vi "Main Page.vi"(8 "error in (no error)":errorcluster, 11 "Node Ptr":T1 format="%.0x") -> (0 "error out":errorcluster)   [LabVIEW 2019, in "MD4Logger System Explorer.lvlib"]
uses:
  MD4Logger System Explorer.lvlib
  <vilib>/NI VeriStand/Custom Device API/Custom Device Item Ref.ctl
  <vilib>/NI VeriStand/Custom Device API/Custom Device Channel.ctl
  <vilib>/NI VeriStand/Custom Device API/Custom Device Channel Type.ctl
  Shared/Constants.vi
  <vilib>/NI VeriStand/Custom Device API/Get Item Property (Path).vi
  <vilib>/NI VeriStand/Custom Device API/Get Item Property (String).vi
  <vilib>/NI VeriStand/Custom Device Tools/Custom Device Utility Library/NI VeriStand - Search for Item by GUID.vi
  <vilib>/NI VeriStand/Custom Device API/Set Item Property (String).vi
  <vilib>/NI VeriStand/Custom Device API/Set Item Property (Path).vi
  <vilib>/NI VeriStand/Custom Device API/Custom Device API.lvlib
  <vilib>/NI VeriStand/Custom Device Tools/Custom Device Utility Library/Custom Device Utility Library.lvlib
  Shared/MD4Logger Shared.lvlib
panel:
  in  "File Name":string
  in  "Channel Unit":string
  in  "MDF4 Folder Path":path
  in  "Add":bool
  in  "Channel Name":string
  out "Version":string
  in  "Specific Header":cluster{"Section Name":string}={"Section Name"="Custom Device Item Settings"}
  in  "General Header":cluster{"Section Name":string}={"Section Name"="General Custom Device Settings"}
  in  "Description":string
  in  "Name":string
  # "STEPS\n\nConfiguration\n1. Set the folder path where the MDF4 files should be logged and set the FileName.\n2. Set the Channel Name and Unit and click Add Channel to create MDF4 channels.\n\nRunning\n1. Create New File by setting Command CreateFile to 1\n2. Enable StartLogging by setting Command StartLogging to 1"
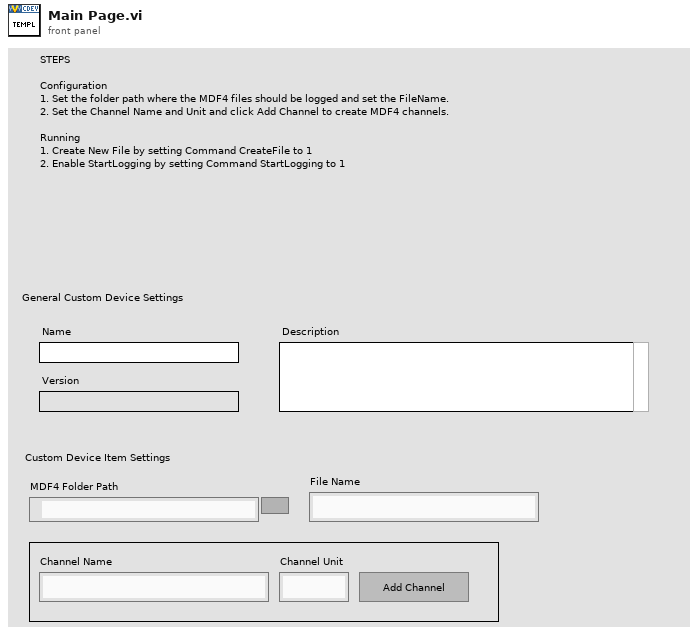
[diagram p1: front panel]
types:
  T1 = typedef "Custom Device API.lvlib/Custom Device Item Ref.ctl" = u64
  T2 = typedef "Custom Device API.lvlib/Custom Device Item Info.ctl" = cluster{"Name":string, "Is Channel":bool, "GUID":string, "Is Waveform":bool}
  T3 = typedef "Custom Device API.lvlib/Custom Device Channel.ctl" = cluster{"Type":T4, "Units":string, "Default Value":dbl, "Faultable":bool, "Scalable":bool}
  T4 = typedef "Custom Device API.lvlib/Custom Device Channel Type.ctl" = enum16{"Input", "Output"}
  T5 = typedef "Custom Device API.lvlib/Custom Device Commands.ctl" = enum16{"Default", "Item renamed", "Shutdown", "Dynamic button pressed"}
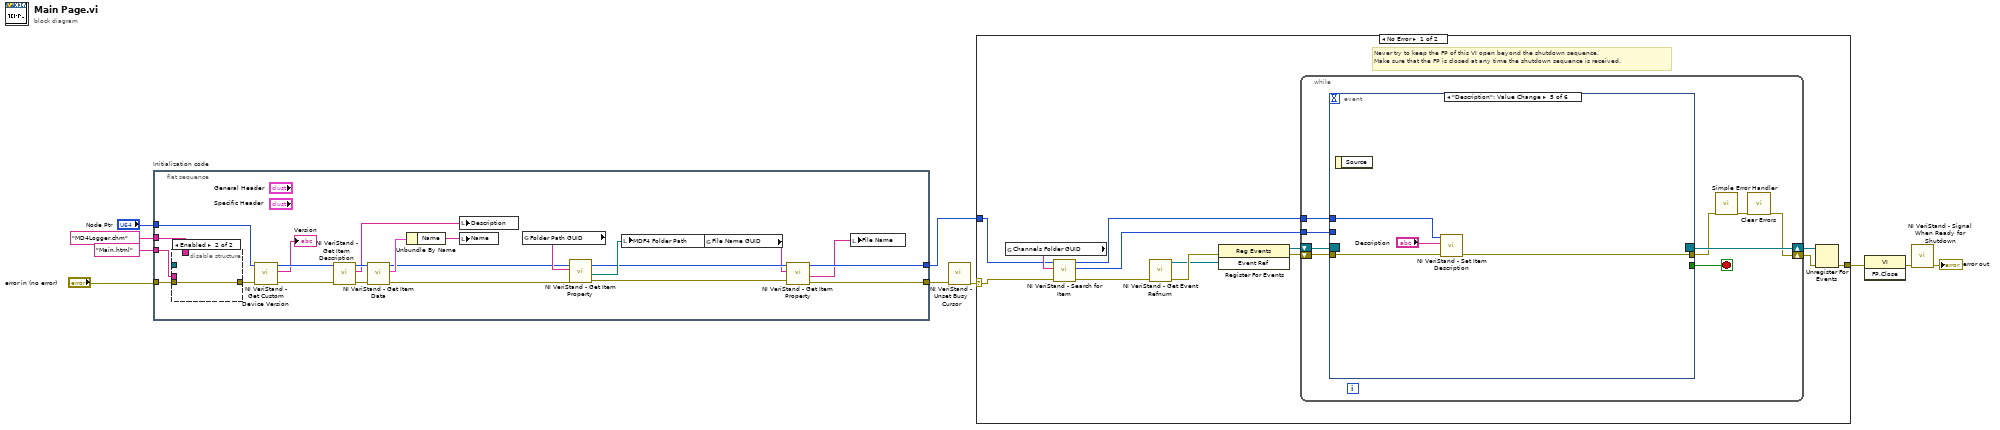
[diagram p0: block diagram]
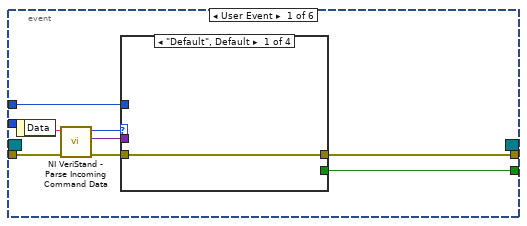
[diagram p2: hidden frame]
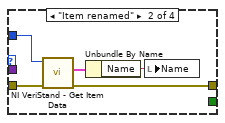
[diagram p3: hidden frame]
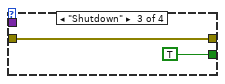
[diagram p4: hidden frame]
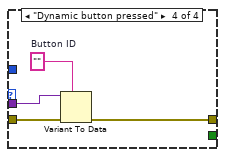
[diagram p5: hidden frame]
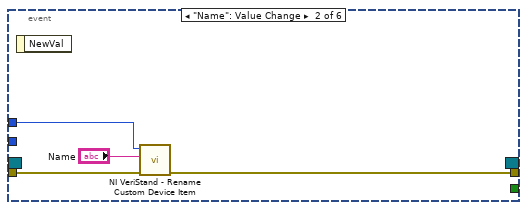
[diagram p6: hidden frame]
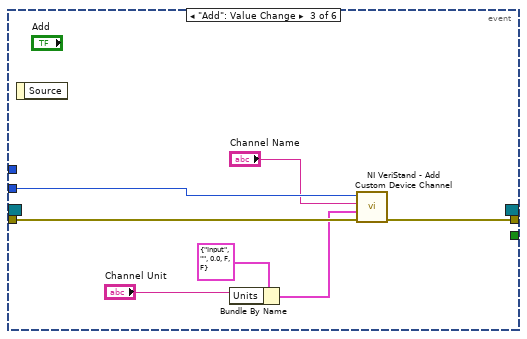
[diagram p7: hidden frame]
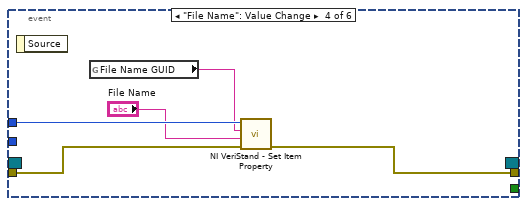
[diagram p8: hidden frame]
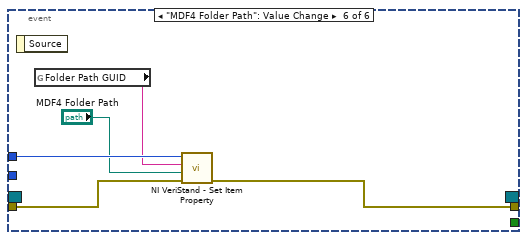
[diagram p9: hidden frame]
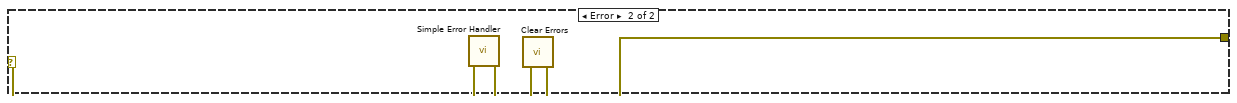
[diagram p10: hidden frame]
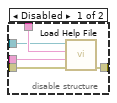
[diagram p11: hidden frame]
diagram:
  n1 = flat-sequence "Initialization code" {
    tunnel: "error in (no error)" -> [w25]
    tunnel: "Node Ptr" -> [w30]
    tunnel: [w14] -> w9
    tunnel: [w13] -> w7
    tunnel: "Main.html" ("HTML File") -> [w24]
    tunnel: "MD4Logger.chm" ("CD_CHM_FileName") -> [w23]
    frame #0 {
      n2 = disable-structure shown="Enabled" {
        disable-tunnel: [w38 w39] -> w26
        disable-tunnel: w25 -> [w37 w39]
        disable-tunnel: w24 -> [w36 _]
        disable-tunnel: w23 -> [w35 _]
        disable-tunnel: _ -> [w34 _]
        frame Disabled {
          n3 = call "Load Help File.vi"("error in (no error)"=w37, "HTML File to Load"=w36, "Main CHM File"=w35, "Browser"=w34) -> ("error out"=w38:errorcluster)  [unwired: 7 in]
        }
        frame Enabled {
        }
      }
      n4 = call <vilib>:"NI VeriStand - Get Custom Device Version.vi"("error in (no error)"=w26, "Device Ref in"=w30) -> ("error out"=w29:errorcluster, "Value"=→"Version":string, "Device Ref out"=w28:T1)  [unwired: 7 in]
      n5 = call <vilib>:"NI VeriStand - Get Item Description.vi"("error in (no error)"=w29, "Item Ref in"=w28) -> ("error out"=w32:errorcluster, "Description"=w21:string, "Item Ref out"=w33:T1)  [unwired: 7 out]
      n6 = call <vilib>:"NI VeriStand - Get Item Data.vi"("error in (no error)"=w32, "Item Ref in"=w33) -> ("error out"=w17:errorcluster, "Item Info"=w31:T2, "Item Ref out"=w18:T1)  [unwired: 7 out]
      n7 = Unbundle By Name(w31) -> ("Name"=w22:string)
      n8 = local write "Description"(w21) -> ()
      n9 = local write "Name"(w22) -> ()
      n10 = global read "Constants.vi" "Folder Path GUID"() -> (w20:string)
      n11 = call-poly <vilib>:"NI VeriStand - Get Item Property.vi"("error in (no error)"=w17, "Property Name"=w20, "Item Ref in"=w18) -> ("error out"=w15:errorcluster, "Value"=w19:path, "Item Ref out"=w16:T1)  [unwired: 5 in, 1 out]
      n12 = local write "MDF4 Folder Path"(w19) -> ()
      n13 = global read "Constants.vi" "File Name GUID"() -> (w12:string)
      n14 = call-poly <vilib>:"NI VeriStand - Get Item Property.vi"("error in (no error)"=w15, "Property Name"=w12, "Item Ref in"=w16) -> ("error out"=w14:errorcluster, "Value"=w11:string, "Item Ref out"=w13:T1)  [unwired: 5 in, 1 out]
      n15 = local write "File Name"(w11) -> ()
    }
  }
  n16 = call <vilib>:"NI VeriStand - Unset Busy Cursor.vi"("error in (no error)"=w9) -> ("error out"=w1:errorcluster)  [unwired: 10 out]
  n17 = case shown="No Error" w1 {
    selector: w1 -> [w43 w109]
    tunnel: [w49 w107] -> w4
    tunnel: w7 -> [w44 _]
    frame No Error {
      # "Never try to keep the FP of this VI open beyond the shutdown sequence.\nMake sure that the FP is closed at any time the shutdown sequence is received."
      n18 = global read "Constants.vi" "Channels Folder GUID"() -> (w45:string)
      n19 = call-poly <vilib>:"NI VeriStand - Search for Item.vi"("error in"=w43, "Item GUID"=w45, "Section Ref in"=w44) -> ("error out"=w42:errorcluster, "Item Ref"=w40:T1, "Section Ref out"=w41:T1)  [unwired: 5 in, 1 out]
      n20 = call <vilib>:"NI VeriStand - Get Event Refnum.vi"("error in (no error)"=w42) -> ("error out"=w52:errorcluster, "Event Ref"=w48:refnum<user-event>)  [unwired: 9 out]
      n21 = register-events(error in=w52, w48) -> (reference out=w46:refnum<event-registration>, error out=w47:errorcluster)  [unwired: 1 in]
      n22 = while {
        tunnel: w41 -> [w57]
        shift-right: [w54] -> w50
        shift-left: w47 -> [w60]
        shift-right: [w61] -> w51
        shift-left: w46 -> [w59]
        tunnel: w40 -> [w53]
        stop <- w58 stop-if-true
        n23 = event shown="[4] \"Description\": Value Change" {
          selector: w59 -> [_ _ _ _ _ _]
          dyn-events: [_ _ _ _ _ _] -> w61
          timeout: _ -> [_ _ _ _ _ _]
          tunnel: w60 -> [w69 w85 w91 w94 w100 w104]
          tunnel: [w65 _ _ _ _ _] -> w58
          tunnel: [w64 w84 w89 w93 w99 w105] -> w56
          tunnel: w57 -> [w63 w83 _ w97 w101 w106]
          tunnel: w53 -> [_ _ w92 _ _ _]
          event User Event {
            n24 = event-data() -> ("Data"=w68:string)  [unwired: 1 out]
            n25 = call <vilib>:"NI VeriStand - Parse Incoming Command Data.vi"("error in (no error)"=w69, "Incoming data"=w68) -> ("error out"=w67:errorcluster, "Outgoing data"=w62:variant, "Action"=w66:T5)  [unwired: 7 out]
            n26 = case shown="\"Default\", Default" w66 {
              tunnel: w67 -> [w70 w75 w76 w81]
              tunnel: [_ _ TRUE _] -> w65
              tunnel: [w70 w72 w76 w78] -> w64
              tunnel: w63 -> [_ w74 _ _]
              tunnel: w62 -> [_ _ _ w80]
              frame "Default", Default {
              }
              frame "Item renamed" {
                n27 = call <vilib>:"NI VeriStand - Get Item Data.vi"("error in (no error)"=w75, "Item Ref in"=w74) -> ("error out"=w72:errorcluster, "Item Info"=w73:T2)  [unwired: 8 out]
                n28 = Unbundle By Name(w73) -> ("Name"=w71:string)
                n29 = local write "Name"(w71) -> ()
              }
              frame "Shutdown" {
              }
              frame "Dynamic button pressed" {
                w79 = ""  # Button ID
                n30 = Variant To Data(error in=w81, type=w79, Variant=w80) -> (error out=w78:errorcluster)  [unwired: 1 out]
              }
            }
          }
          event "Name": Value Change {
            n31 = event-data() -> ()  [unwired: 2 out]
            n32 = call <vilib>:"NI VeriStand - Rename Custom Device Item.vi"("error in (no error)"=w85, "New Name"="Name", "Item Ref in"=w83) -> ("error out"=w84:errorcluster)  [unwired: 1 in, 7 out]
          }
          event "Add": Value Change {
            n33 = event-data() -> ()  [unwired: 2 out]
            n34 = Bundle By Name(cluster=T3 {"Type"=enum."Input", "Units"="", "Default Value"=0.0, "Faultable"=FALSE, "Scalable"=FALSE} ("Channel"), "Units"="Channel Unit") -> (w86:T3)
            n35 = call <vilib>:"NI VeriStand - Add Custom Device Channel.vi"("error in (no error)"=w91, "Channel"=w86, "Channel Name"="Channel Name", "Parent Ref in"=w92) -> ("error out"=w89:errorcluster)  [unwired: 4 in, 3 out]
          }
          event "File Name": Value Change {
            n36 = event-data() -> ()  [unwired: 2 out]
            n37 = global read "Constants.vi" "File Name GUID"() -> (w96:string)
            n38 = call-poly <vilib>:"NI VeriStand - Set Item Property.vi"("error in (no error)"=w94, "Value"="File Name", "Property Name"=w96, "Item Ref in"=w97) -> ("error out"=w93:errorcluster)  [unwired: 5 in, 2 out]
          }
          event "Description": Value Change {
            n39 = event-data() -> ()  [unwired: 2 out]
            n40 = call <vilib>:"NI VeriStand - Set Item Description.vi"("error in (no error)"=w100, "Description"="Description", "Item Ref in"=w101) -> ("error out"=w99:errorcluster)  [unwired: 8 out]
          }
          event "MDF4 Folder Path": Value Change {
            n41 = event-data() -> ()  [unwired: 2 out]
            n42 = global read "Constants.vi" "Folder Path GUID"() -> (w102:string)
            n43 = call-poly <vilib>:"NI VeriStand - Set Item Property.vi"("error in (no error)"=w104, "Value"="MDF4 Folder Path", "Property Name"=w102, "Item Ref in"=w106) -> ("error out"=w105:errorcluster)  [unwired: 5 in, 2 out]
          }
        }
        n44 = call <vilib>:"Simple Error Handler.vi"("error in (no error)"=w56) -> ("error out"=w55:errorcluster)  [unwired: 1 in, 7 out]
        n45 = call <vilib>:"Clear Errors.vi"("error in (no error)"=w55) -> ("error out"=w54:errorcluster)  [unwired: 1 in, 5 out]
      }
      n46 = Unregister For Events(event registration refnum=w51, error in=w50) -> (error out=w49:errorcluster)
    }
    frame Error {
      n47 = call <vilib>:"Simple Error Handler.vi"("error in (no error)"=w109) -> ("error out"=w108:errorcluster)  [unwired: 1 in, 7 out]
      n48 = call <vilib>:"Clear Errors.vi"("error in (no error)"=w108) -> ("error out"=w107:errorcluster)  [unwired: 1 in, 5 out]
    }
  }
  n49 = invoke class="VI" method="FP.Close"(error in=w4) -> (error out=w3:errorcluster)  [unwired: 2 in, 2 out]
  n50 = call <vilib>:"NI VeriStand - Signal When Ready for Shutdown.vi"("error in (no error)"=w3) -> ("error out"=→"error out":errorcluster)  [unwired: 10 out]
